vi "fgv_232_F9P.vi"(7 "cmd":enum16{"init", "read", "write", "close"}(ring), 8 "error in":errorcluster, 10 "write buff":string) -> (0 "error out":errorcluster, 3 "read_buffer":string)   [LabVIEW 2019]
uses:
  <vilib>/Instr/_visa.llb/VISA Configure Serial Port (Instr).vi
panel:
  out "Waveform Chart":u32(graph)
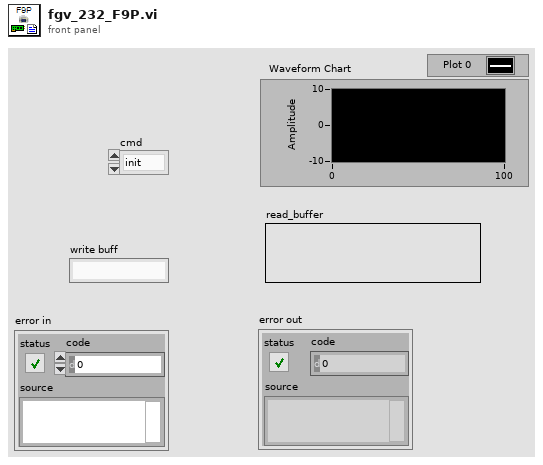
[diagram p1: front panel]
types:
  T1 = cluster{"Port":refnum<visa-resource-name>, "heading select":string, "mode select":string[]}
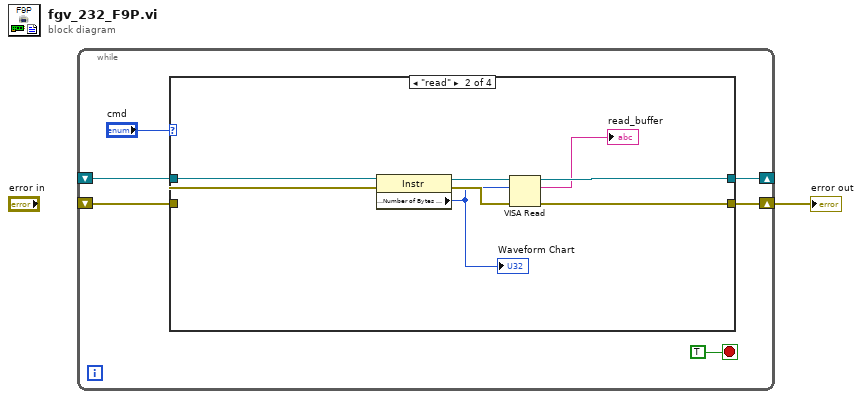
[diagram p0: block diagram]
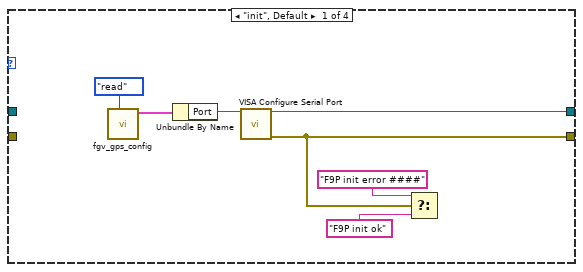
[diagram p2: hidden frame]
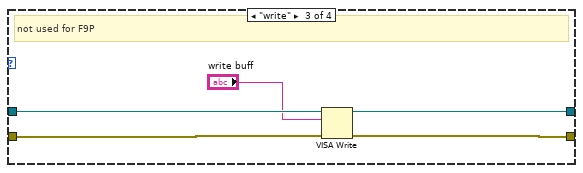
[diagram p3: hidden frame]
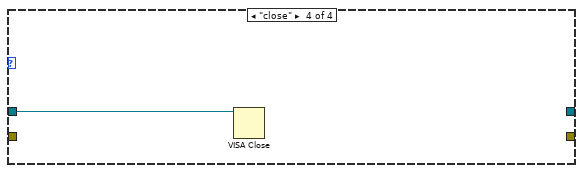
[diagram p4: hidden frame]
diagram:
  n1 = while {
    shift-right: [w5] -> _
    shift-left: _ -> [w3]
    shift-right: [w4] -> w1
    shift-left: _ -> [w2]
    stop <- TRUE stop-if-true
    n2 = case shown="\"read\"" "cmd" {
      tunnel: [w14 w20 w25 _] -> w5
      tunnel: [w13 w19 w24 _] -> w4
      tunnel: w3 -> [_ w22 w26 w28]
      tunnel: w2 -> [_ w17 w27 _]
      frame "init", Default {
        n3 = call "fgv_gps_config.vi"("cmd"=enum16{"read", "write"}."read") -> ("cfg out"=w9:T1)  [unwired: 9 in, 1 out]
        n4 = Unbundle By Name(w9) -> ("Port"=w8:refnum<visa-resource-name>)
        n5 = call-poly "VISA Configure Serial Port"("VISA resource name"=w8) -> ("VISA resource name out"=w14:refnum<visa-resource-name>, "error out"=w13:errorcluster)  [unwired: 13 in]
        n6 = Select(t="F9P init error ####" ("String in"), s=w13, f="F9P init ok" ("String in")) -> ()  [unwired: 1 out]
      }
      frame "read" {
        n7 = property class="Instr"(reference=w22, error in=w17) -> (reference out=w21:refnum<visa-resource-name>, error out=w18:errorcluster, "Serial Settings:Number of Bytes at Serial Port"=w15:u32)
        "Waveform Chart" <- w15
        n8 = VISA Read(VISA resource name=w21, byte count=w15, error in (no error)=w18) -> (VISA resource name out=w20:refnum<visa-resource-name>, read buffer=→"read_buffer":string, error out=w19:errorcluster)  [unwired: 1 out]
      }
      frame "write" {
        # "not used for F9P"
        n9 = VISA Write(VISA resource name=w26, write buffer="write buff", error in (no error)=w27) -> (VISA resource name out=w25:refnum<visa-resource-name>, error out=w24:errorcluster)  [unwired: 1 out]
      }
      frame "close" {
        n10 = VISA Close(VISA resource name=w28) -> ()  [unwired: 1 in, 1 out]
      }
    }
  }
  "error out" <- w1
